vi "LedTest.vi"() -> ()   [LabVIEW 2020]
panel:
  in  "Red/Green [T/F]":bool
  in  "Stop Button":bool
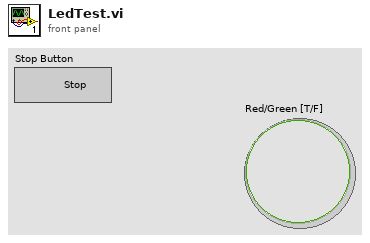
[diagram p1: front panel]
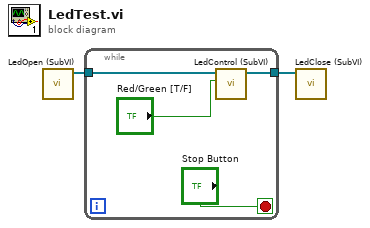
[diagram p0: block diagram]
diagram:
  n1 = call "LedOpen (SubVI).vi"() -> ("LedRef"=w2:refnum<class "Digital Output.lvclass">[])  [unwired: 10 in, 1 out]
  n2 = while {
    tunnel: w2 -> [w5]
    tunnel: [w3] -> w1
    stop <- "Stop Button" stop-if-true
    n3 = call "LedControl (SubVI).vi"("Red/Green [T/F]"="Red/Green [T/F]", "LedRef"=w5) -> ("LedRef"=w3:refnum<class "Digital Output.lvclass">[])  [unwired: 8 in, 1 out]
  }
  n4 = call "LedClose (SubVI).vi"("LedRef"=w1) -> ()  [unwired: 10 in, 1 out]
